vi "Serialize.vi"(8 "error in (no error)":errorcluster, 10 "Element in":refnum<k20>, 11 "Test Case in":refnum<class "Test Case.lvclass">) -> (0 "error out":errorcluster, 2 "Element out":refnum<k20>)   [LabVIEW 2013, in "JUnit XML.lvlib" / "Test Case.lvclass"]
doc: "Serializes a Test Case using NI XML Parser."
uses:
  Test Case.lvclass
  Test Case.lvclass/Test Case.ctl
  <vilib>/xml/Close Reference(Node).vi
  <vilib>/xml/NI_XML.lvlib
  JUnit XML.lvlib
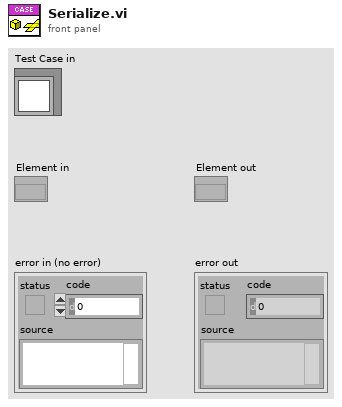
[diagram p1: front panel]
types:
  T1 = typedef "JUnit XML.lvlib/Test Case.lvclass/Test Result.ctl" = enum16{"Success", "Failure", "Error", "Skipped"}
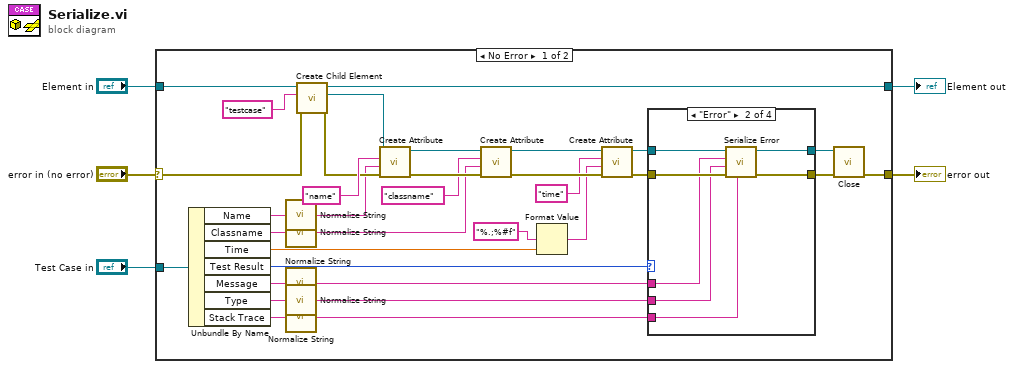
[diagram p0: block diagram]
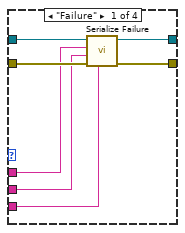
[diagram p2: hidden frame]
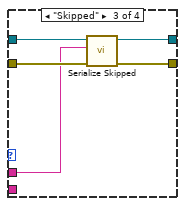
[diagram p3: hidden frame]
diagram:
  n1 = case shown="No Error" "error in (no error)" {
    selector: "error in (no error)" -> [w15 w61]
    tunnel: [w14 w61] -> w4
    tunnel: "Test Case in" -> [w13 _]
    tunnel: "Element in" -> [w12 w60]
    tunnel: [w11 w60] -> w1
    frame No Error {
      n2 = Unbundle By Name(w13) -> ("Name"=w36:string, "Classname"=w26:string, "Time"=w25:dbl, "Test Result"=w23:T1, "Message"=w20:string, "Type"=w19:string, "Stack Trace"=w16:string)
      n3 = call "Normalize String.vi"("String"=w36) -> ("Normalized String"=w10:string)  [unwired: 1 in]
      n4 = call "Normalize String.vi"("String"=w26) -> ("Normalized String"=w9:string)  [unwired: 1 in]
      n5 = call "Normalize String.vi"("String"=w20) -> ("Normalized String"=w7:string)  [unwired: 1 in]
      n6 = call "Normalize String.vi"("String"=w19) -> ("Normalized String"=w8:string)  [unwired: 1 in]
      n7 = call "Normalize String.vi"("String"=w16) -> ("Normalized String"=w6:string)  [unwired: 1 in]
      n8 = call "Create Child Element.vi"("error in (no error)"=w15, "Name"="testcase" ("Tag Name"), "Element in"=w12) -> ("error out"=w27:errorcluster, "Child Element"=w28:refnum<k20>, "Element out"=w11:refnum<k20>)  [unwired: 6 in]
      n9 = call "Create Attribute.vi"("error in (no error)"=w27, "Value"=w10, "Name"="name" ("Attribute Name"), "Element in"=w28) -> ("error out"=w34:errorcluster, "Element out"=w35:refnum<k20>)  [unwired: 6 in]
      n10 = call "Create Attribute.vi"("error in (no error)"=w34, "Value"=w9, "Name"="classname" ("Attribute Name"), "Element in"=w35) -> ("error out"=w31:errorcluster, "Element out"=w32:refnum<k20>)  [unwired: 6 in]
      n11 = Format Value(format string="%.;%#f", value (0)=w25) -> (output string=w24:string)  [unwired: 1 in]
      n12 = call "Create Attribute.vi"("error in (no error)"=w31, "Value"=w24, "Name"="time" ("Attribute Name"), "Element in"=w32) -> ("error out"=w17:errorcluster, "Element out"=w18:refnum<k20>)  [unwired: 6 in]
      n13 = case shown="\"Error\"" w23 {
        tunnel: w18 -> [w45 w52 w57 w59]
        tunnel: [w44 w51 w56 w59] -> w22
        tunnel: [w43 w50 w55 w58] -> w21
        tunnel: w17 -> [w42 w49 w54 w58]
        tunnel: w7 -> [w41 w48 w53 _]
        tunnel: w8 -> [w40 w47 _ _]
        tunnel: w6 -> [w39 w46 _ _]
        frame "Failure" {
          n14 = call "Serialize Failure.vi"("Stack Trace"=w39, "error in (no error)"=w42, "Type"=w40, "Message"=w41, "Node in"=w45) -> ("error out"=w43:errorcluster, "Node out"=w44:refnum<k20>)  [unwired: 5 in]
        }
        frame "Error" {
          n15 = call "Serialize Error.vi"("Stack Trace"=w46, "error in (no error)"=w49, "Type"=w47, "Message"=w48, "Node in"=w52) -> ("error out"=w50:errorcluster, "Node out"=w51:refnum<k20>)  [unwired: 5 in]
        }
        frame "Skipped" {
          n16 = call "Serialize Skipped.vi"("error in (no error)"=w54, "Message"=w53, "Node in"=w57) -> ("error out"=w55:errorcluster, "Node out"=w56:refnum<k20>)  [unwired: 7 in]
        }
        frame "Success" {
        }
      }
      n17 = call-poly <vilib>:"Close.vi"("error in (no error)"=w21, "node"=w22) -> ("error out"=w14:errorcluster)  [unwired: 7 in]
    }
    frame Error {
    }
  }
  "error out" <- w4
  "Element out" <- w1
